vi "SetDefault.vi"(7 "error in (no error)":errorcluster, 9 "Default Autonomous Mode":string, 10 "Table Prefix":string="330AutonomousSelector") -> (0 "error out":errorcluster)   [LabVIEW 2015, in "BB_AutonomousSelector.lvlib"]
doc: "Sets the default Autonomous Mode. This adds the Autonomous Mode if it wasn't already added. It sets the selected Autonomous Mode on the dashboard until the user overrides it. If no Autonomous Mode is selected on the Dashboard, the default is used. \n\n<B>Table Prefix</B> The Sub Table in Network Tables. The data will be stored in /SmartDashboard/<Table Prefix>\n<B>Default</B> The Autonomous Mode to use as default."
uses:
  BB_AutonomousSelector.lvlib
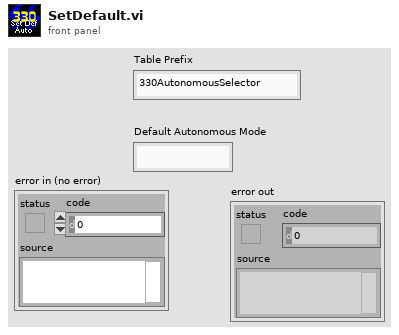
[diagram p1: front panel]
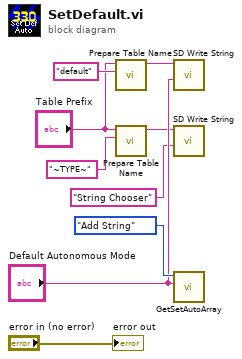
[diagram p0: block diagram]
diagram:
  n1 = call <vilib>:"Prepare Table Name.vi"("Name"="default", "Table Prefix"="Table Prefix") -> ("Prefixed Name"=w8:string)  [unwired: 9 in]
  n2 = call <vilib>:"Prepare Table Name.vi"("Name"="~TYPE~", "Table Prefix"="Table Prefix") -> ("Prefixed Name"=w1:string)  [unwired: 9 in]
  n3 = call <vilib>:"SD Write String.vi"("String"="Default Autonomous Mode", "Name"=w8) -> ()  [unwired: 8 in, 2 out]
  n4 = call <vilib>:"SD Write String.vi"("String"="String Chooser", "Name"=w1) -> ()  [unwired: 8 in, 2 out]
  n5 = call "GetSetAutoArray.vi"("String"="Default Autonomous Mode", "Mode"=enum16{"Get", "Add String", "Add String Array"}."Add String") -> ()  [unwired: 9 in, 1 out]
  "error out" <- "error in (no error)"
